vi "add_point.vi"(8 "error in (no error)":errorcluster, 10 "point (x/y/z)":dbl[](array[numeric]), 11 "PointCollection in":refnum<class "PointCollection.lvclass">) -> (0 "error out":errorcluster, 3 "PointCollection out":refnum<class "PointCollection.lvclass">)   [LabVIEW 2010, in "PointCollection.lvclass"]
uses:
  PointCollection.lvclass
  mode_enum.ctl
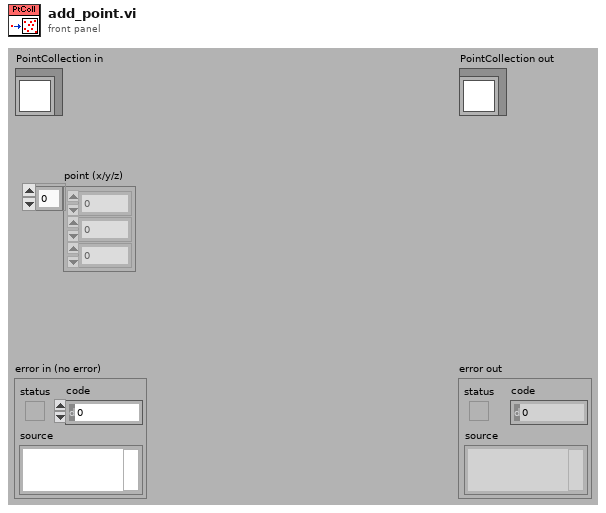
[diagram p1: front panel]
types:
  T1 = typedef "PointCollection.lvclass/mode_enum.ctl" = enum16{"points first", "dimensions first"}
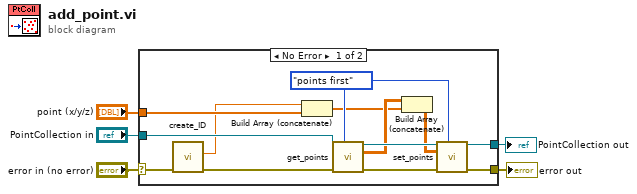
[diagram p0: block diagram]
diagram:
  n1 = case shown="No Error" "error in (no error)" {
    selector: "error in (no error)" -> [w9 w20]
    tunnel: [w17 w20] -> w4
    tunnel: [w15 w19] -> w2
    tunnel: "PointCollection in" -> [w7 w19]
    tunnel: "point (x/y/z)" -> [w11 _]
    frame No Error {
      w12 = mode_enum."points first" ("retrieval mode")
      n2 = call "create_ID.vi"("error in (no error)"=w9) -> ("error out"=w8:errorcluster, "ID"=w6:dbl)  [unwired: 9 in]
      n3 = Build Array (concatenate)(w6, w11) -> (w10:dbl[])
      n4 = call-dynamic "get_points.vi"("retrieval mode"=w12, "error in (no error)"=w8, "PointCollection in"=w7) -> ("error out"=w18:errorcluster, "points"=w14:dbl[][], "PointCollection out"=w16:refnum<class "PointCollection.lvclass">)  [unwired: 6 in]
      n5 = Build Array (concatenate)(w14, w10) -> (w13:dbl[][])
      n6 = call "set_points.vi"("mode"=w12, "error in (no error)"=w18, "points (dimensions/points)"=w13, "PointCollection in"=w16) -> ("error out"=w17:errorcluster, "PointCollection out"=w15:refnum<class "PointCollection.lvclass">)  [unwired: 6 in]
    }
    frame Error {
    }
  }
  "error out" <- w4
  "PointCollection out" <- w2
